vi "Sync Config from Instr.vi"(8 "error in (no error)":errorcluster, 11 "LakeShore T Controller Driver in":refnum<class "LakeShore T Controller Driver.lvclass">) -> (0 "error out":errorcluster, 2 "Variant":variant, 3 "LakeShore T Controller Driver out":refnum<class "LakeShore T Controller Driver.lvclass">)   [LabVIEW 2024, in "LakeShore T Controller Driver.lvclass"]
uses:
  LakeShore T Controller Driver.lvclass
  VISA Instrument/VISA Instrument.lvclass/VISA Instrument.ctl
  VISA Instrument/Read VISA resource.vi
  VISA Instrument/Write VISA resource.vi
  Temperature Controller Driver/Read T controller configuration.vi
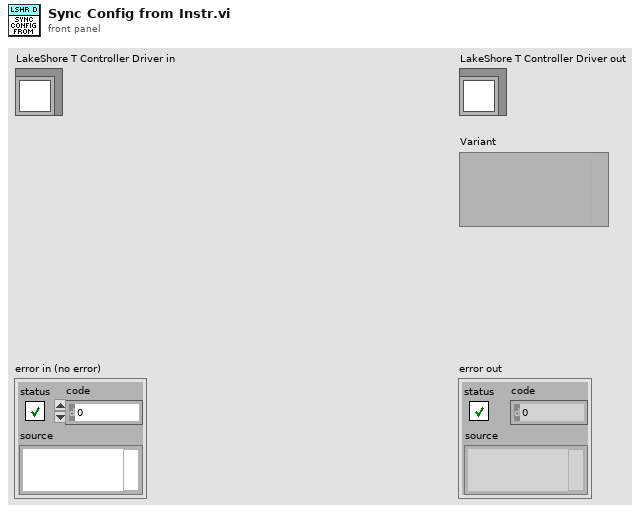
[diagram p1: front panel]
types:
  T1 = typedef "T controller configuration.ctl" = cluster{"Record Channels":string[], "Record raw signal":bool, "Set point":dbl, "Record heater":bool, "Ramp rate":dbl, "P":dbl, "I":dbl, "D":dbl, "Control":T2, "P manual":dbl, "Output #":i32}
  T2 = typedef "Control Mode.ctl" = enum16{"Off", "PID", "Ramp", "Manual", "Table"}
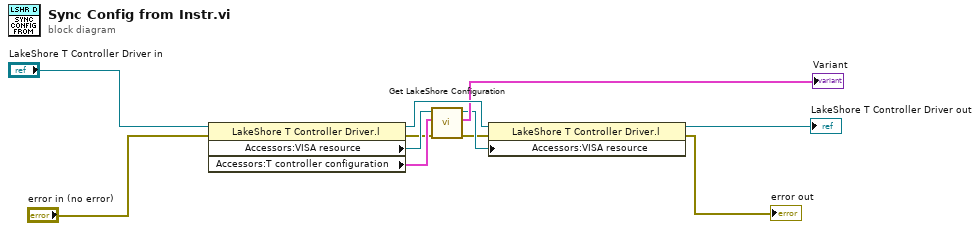
[diagram p0: block diagram]
diagram:
  n1 = property class="LakeShore T Controller Driver.l"(reference="LakeShore T Controller Driver in", error in="error in (no error)") -> (reference out=w10:refnum<class "LakeShore T Controller Driver.lvclass">, error out=w4:errorcluster, "Accessors:VISA resource"=w8:refnum<visa-resource-name>, "Accessors:T controller configuration"=w7:T1)
  n2 = call "Get LakeShore Configuration.vi"("error in (no error)"=w4, "Config in"=w7, "VISA Resource Name"=w8) -> ("error out"=w3:errorcluster, "Config out"=→"Variant":T1, "VISA Resource Name Out"=w5:refnum<visa-resource-name>)  [unwired: 6 in]
  n3 = property class="LakeShore T Controller Driver.l"(reference=w10, error in=w3, "Accessors:VISA resource"=w5) -> (reference out=→"LakeShore T Controller Driver out":refnum<class "LakeShore T Controller Driver.lvclass">, error out=→"error out":errorcluster)
